vi "End Message.vi"(8 "Error In":errorcluster, 9 "Reset ID On Browser? (false)":bool, 10 "Message ID (blank)":string, 11 "Message In":string) -> (0 "Error Out":errorcluster, 3 "Message Out":string)   [LabVIEW 2014, in "i3-sse-server.lvlib"]
uses:
  i3-sse-server.lvlib
  <vilib>/Utility/error.llb/Error Cluster From Error Code.vi
  <vilib>/ErrorRing/Error Ring.xnode
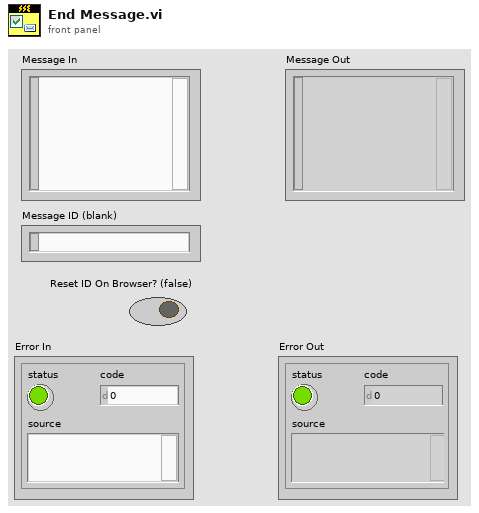
[diagram p1: front panel]
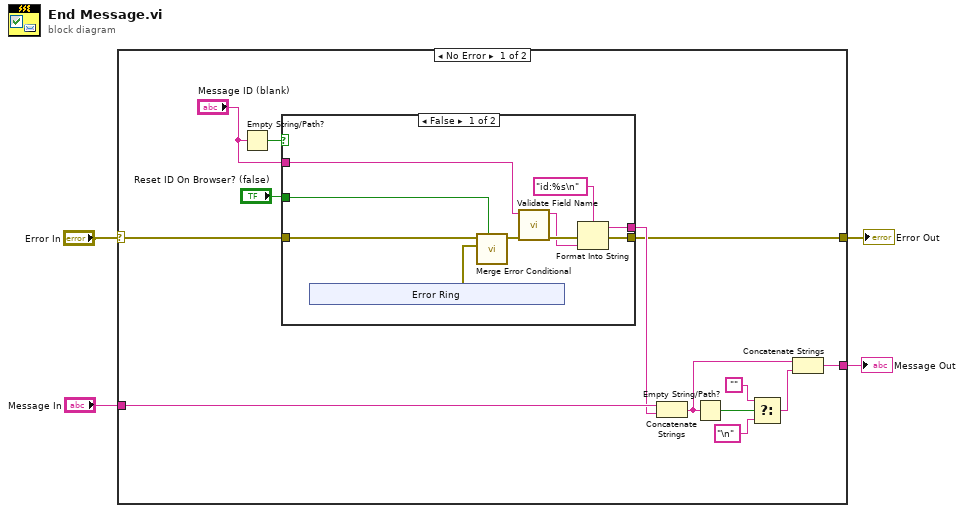
[diagram p0: block diagram]
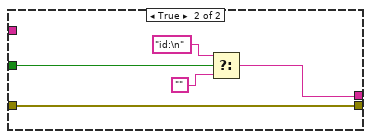
[diagram p2: hidden frame]
diagram:
  n1 = case shown="No Error" "Error In" {
    selector: "Error In" -> [w14 w39]
    tunnel: [w12 w39] -> w2
    tunnel: [w5 w38] -> w3
    tunnel: "Message In" -> [w17 w38]
    frame No Error {
      n2 = Empty String/Path?(string/path="Message ID (blank)") -> (empty?=w16:bool)
      n3 = case shown="False" w16 {
        tunnel: "Message ID (blank)" -> [w24 _]
        tunnel: w14 -> [w20 w37]
        tunnel: [w26 w37] -> w12
        tunnel: [w27 w34] -> w13
        tunnel: "Reset ID On Browser? (false)" -> [w19 w36]
        frame False {
          n4 = xnode "Error Ring"() -> ("error out"=w18:errorcluster)
          n5 = call "Merge Error Conditional.vi"("Merge Error? (true)"=w19, "Error To Merge"=w18, "Original Error Wire"=w20) -> ("Error Out"=w21:errorcluster)  [unwired: 8 in]
          n6 = call "Validate Field Name.vi"("Error In"=w21, "Field Name In"=w24) -> ("Error Out"=w25:errorcluster, "Field Name Out"=w23:string)  [unwired: 8 in]
          n7 = Format Into String(format string="id:%s\n", error in=w25, w23) -> (resulting string=w27:string, error out=w26:errorcluster)  [unwired: 1 in]
        }
        frame True {
          n8 = Select(t="id:\n", s=w36, f="") -> (s? t:f=w34:string)
        }
      }
      n9 = Concatenate Strings(w17, w13) -> (w8:string)
      n10 = Empty String/Path?(string/path=w8) -> (empty?=w10:bool)
      n11 = Select(t="", s=w10, f="\n" ("string")) -> (s? t:f=w6:string)
      n12 = Concatenate Strings(w8, w6) -> (w5:string)
    }
    frame Error {
    }
  }
  "Error Out" <- w2
  "Message Out" <- w3
